vi "ConvertToHTMLPostamble.vi"(0 "ROS in":T1, 1 "Text to add":string) -> (2 "String":string)   [LabVIEW 2012]
uses:
  <userlib>/ROSforLV/ROS/Code/SubVIs/_ROSControl.ctl
  <userlib>/ROSforLV/ROS/Code/SubVIs/_ROSDirection.ctl
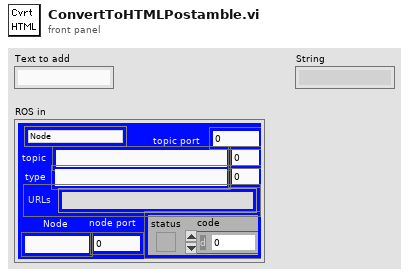
[diagram p1: front panel]
types:
  T1 = typedef "_ROSControl.ctl" = cluster{"topic port":u16, "Node":string, "topic":string, "type":string, "node port":u16, "error ":errorcluster, "Direction":T2, "APIs":string[], "Update (ms)":u16, "write queue":u16}
  T2 = typedef "_ROSDirection.ctl" = enum16{"Node", "Publisher", "Subscriber", "Service Client"}
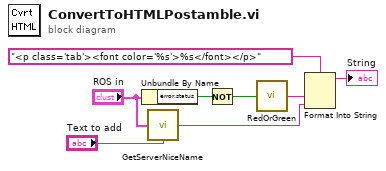
[diagram p0: block diagram]
diagram:
  n1 = Unbundle By Name("ROS in") -> ("error.status"=w3:bool)
  n2 = call <userlib>:"GetServerNiceName.vi"("ROS"="ROS in", "Text to add"="Text to add") -> ("String"=w5:string)
  n3 = Not(x=w3) -> (.not. x?=w1:bool)
  n4 = call <userlib>:"RedOrGreen.vi"("success"=w1) -> ("color"=w4:string)
  n5 = Format Into String(format string="<p class='tab'><font color='%s'>%s</font></p>" ("Text to add"), w4, w5) -> (resulting string=→"String":string)  [unwired: 2 in, 1 out]
